vi "Strain Measurement Data.vi"() -> (0 "Strain-Electrical Measurement":T1={"Configuration"={"Stress Sequence "={"Max Motor Position"=1380.0, "# Intermediate Points"=5000, "Initial Direction"=enum."Tension"}, "Track?"=FALSE}, "Refnums"={"Instrument Steps"=refnum, "Sequence Progress"=refnum, "Device ID"=refnum, "Device Information"=refnum, "Pause-Resume"=refnum, "Track"=refnum, "Plot"={"Plot List"=refnum, "Voltage Plot"=refnum, "Current Plot"=refnum, "IV Characteristic"=refnum, "dI/dV-V Characteristic"=refnum}}} {"Configuration"."Stress Sequence"."# Intermediate Points" max=1390})   [LabVIEW 2014]
uses:
  Strain Measurement Data.ctl
  Strain Measurement Config.ctl
  Strain Measurement Refnums.ctl
  Instrument Sequence/Action.ctl
  Instrument Sequence/Instrument List.ctl
  Plot Data/Electrical Data Plot Refnums.ctl
panel:
  # "LICENSED MATERIALS – PROPERTY OF IBM\nCopyright IBM Corp. 2016,\nALL RIGHTS RESERVED"
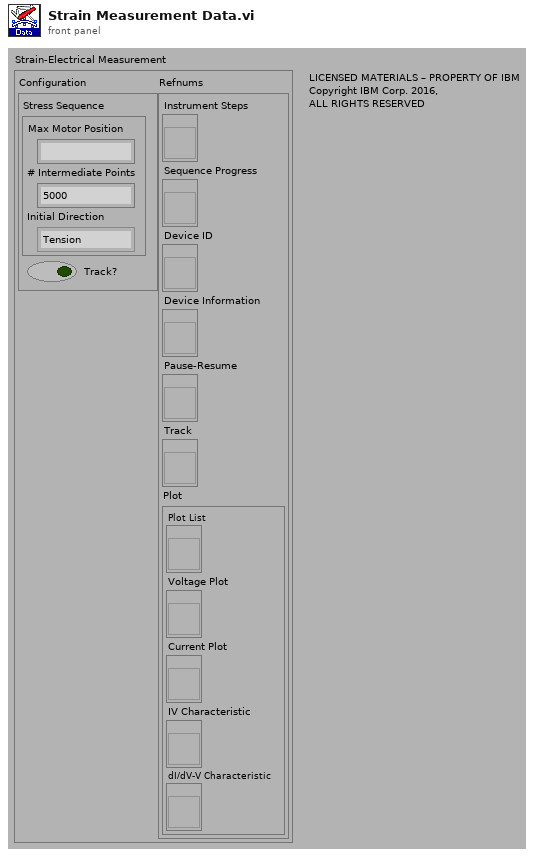
[diagram p1: front panel]
types:
  T1 = typedef "Strain Measurement Data.ctl" = cluster{"Configuration":T2, "Refnums":T3}
  T2 = typedef "Strain Measurement Config.ctl" = cluster{"Stress Sequence ":cluster{"Max Motor Position":ext, "# Intermediate Points":u32, "Initial Direction":enum16{"Tension", "Compression"}}, "Track?":bool}
  T3 = typedef "Strain Measurement Refnums.ctl" = cluster{"Instrument Steps":refnum<vi>, "Sequence Progress":refnum<vi>, "Device ID":refnum<vi>, "Device Information":refnum<vi>, "Pause-Resume":refnum<vi>, "Track":refnum<vi>, "Plot":T4}
  T4 = typedef "Electrical Data Plot Refnums.ctl" = cluster{"Plot List":refnum<vi>, "Voltage Plot":refnum<vi>, "Current Plot":refnum<vi>, "IV Characteristic":refnum<vi>, "dI/dV-V Characteristic":refnum<vi>}
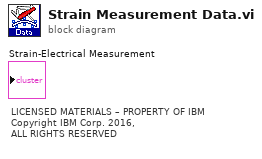
[diagram p0: block diagram]
diagram:
  # "LICENSED MATERIALS – PROPERTY OF IBM\nCopyright IBM Corp. 2016,\nALL RIGHTS RESERVED"
